vi "Manual Control.vi"() -> ()   [LabVIEW 2022 SP3]
uses:
  HMP4000 Communication/HMP4040_ChannelControlAutomatic.ctl
  <vilib>/DAQmx/write.llb/DAQmx Write (Digital Bool 1Line 1Point).vi
  <vilib>/DAQmx/miscellaneous.llb/DAQmx Fill In Error Info.vi
panel:
  in  "stop":bool
  in  "data":bool
  out "HMP VISA Out":refnum<visa-resource-name> caption="VISA resource name out"
  in  "HMP VISA":refnum<visa-resource-name>
  in  "error in (no error)":errorcluster
  in  "Enum":T1
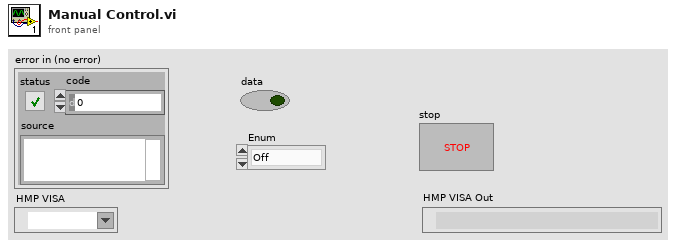
[diagram p1: front panel]
types:
  T1 = typedef "HMP4040_ChannelControlAutomatic.ctl" = enum16{"Off", "Control Power", "HMP2020 Control + DC32V", "HMP2020 Control + DC8V", "HMP4040 Control + DC32V", "HMP4040 Control +DC8V", "HMP4040 Ch2 24V 4A"}
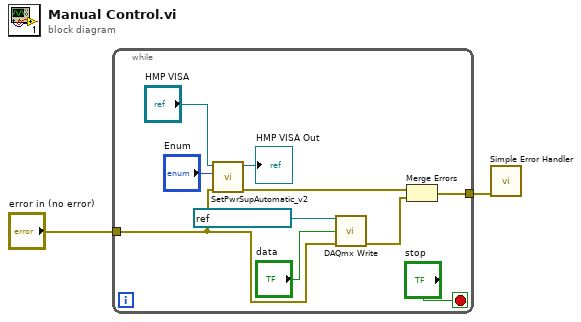
[diagram p0: block diagram]
diagram:
  n1 = while {
    tunnel: "error in (no error)" -> [w6]
    tunnel: [w3] -> w1
    stop <- "stop" stop-if-true
    n2 = call "SetPwrSupAutomatic_v2.vi"("error in (no error)"=w6, "Enum"="Enum", "HMP VISA"="HMP VISA") -> ("error out"=w5:errorcluster, "HMP VISA Out"=→"HMP VISA Out":refnum<visa-resource-name>)  [unwired: 7 in]
    n3 = call-poly <vilib>:"DAQmx Write.vi"("task/channels in"=refnum<k21> "FTS2_120VAC", "data"="data", "error in"=w6) -> ("error out"=w4:errorcluster)  [unwired: 10 in, 2 out]
    n4 = Merge Errors(w5, w4) -> (w3:errorcluster)
  }
  n5 = call <vilib>:"Simple Error Handler.vi"("error in (no error)"=w1) -> ()  [unwired: 4 in, 5 out]
